vi "btc秘钥探测狗.vi"() -> ()   [LabVIEW 2020]
panel:
  out "非压缩地址":string
  out "压缩地址":string
  out "error out":errorcluster caption="错误输出"
  out "账户信息 2":string[](array[string])
  out "账户信息":string[](array[string])
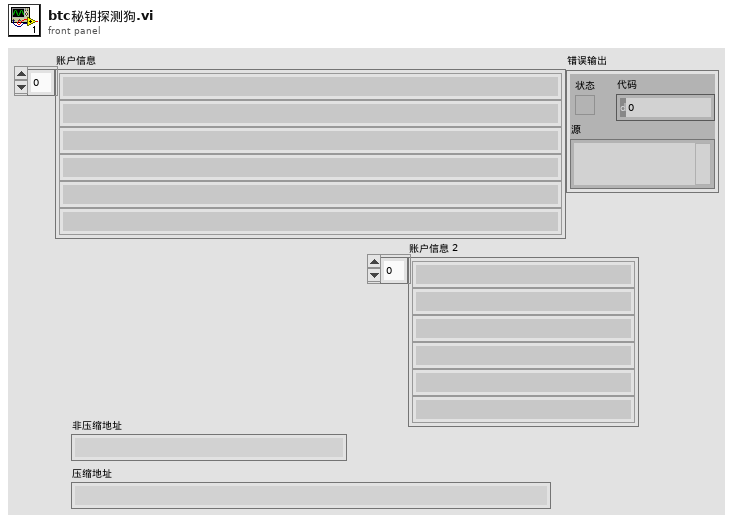
[diagram p1: front panel]
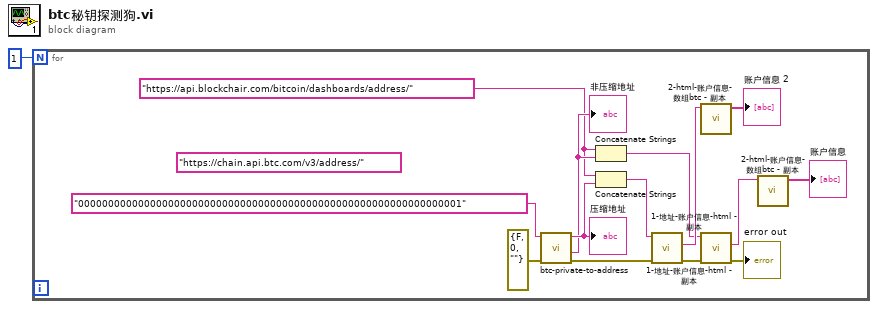
[diagram p0: block diagram]
diagram:
  n1 = for {
    N: 1 -> [_]
    w2 = "https://api.blockchair.com/bitcoin/dashboards/address/" ("URL输入")
    (unwired) "https://chain.api.btc.com/v3/address/" ("URL输入")
    n2 = call "btc-private-to-address.vi"("error in (no error)"=cluster{"状态":bool, "代码":i32, "源":string} {"状态"=FALSE, "代码"=0, "源"=""}, "私钥输入"="0000000000000000000000000000000000000000000000000000000000000001") -> ("error out"=w15:cluster{"状态":bool, "代码":i32, "源":string}, "非压缩地址"=w4:string, "压缩地址"=w6:string)  [unwired: 7 in]
    "压缩地址" <- w6
    "非压缩地址" <- w4
    n3 = Concatenate Strings(w2, w4) -> (w3:string)
    n4 = Concatenate Strings(w2, w6) -> (w5:string)
    n5 = call "1-地址-账户信息-html - 副本.vi"("error in (no error)"=w15, "URL输入"=w5) -> ("error out"=w13:errorcluster, "body"=w14:string)  [unwired: 6 in, 2 out]
    n6 = call "2-html-账户信息-数组btc - 副本.vi"("body"=w14) -> ("账户信息"=→"账户信息 2":string[])  [unwired: 10 in]
    n7 = call "1-地址-账户信息-html - 副本.vi"("error in (no error)"=w13, "URL输入"=w3) -> ("error out"=→"error out":errorcluster, "body"=w12:string)  [unwired: 6 in, 2 out]
    n8 = call "2-html-账户信息-数组btc - 副本.vi"("body"=w12) -> ("账户信息"=→"账户信息":string[])  [unwired: 10 in]
  }
